vi "Custom Photobleach Length.vi"(8 "Stage Limits":T1={"Y Min"=-inf, "Y Max"=inf, "X Min"=-inf, "X Max"=inf}) -> (0 "Canceled":bool, 1 "Speed (µm/s)":dbl, 2 "Lanes":dbl=1.0, 3 "Length (mm)":dbl)   [LabVIEW 2023]
panel:
  in  "Scan Speed (mm/s):":dbl=0.1 min=0.01 max=1.0
  in  "Number of lanes:":dbl=1.0 min=1.0 step=1.0
  in  "Cancel":bool
  in  "OK":bool
  in  "Lane Length (mm):":dbl=6.0 min=1.0 max=8.0 step=1.0
  # "Please confirm that prism is positioned at the far end\nof the lane. Otherwise microscope WILL BE DAMAGED."
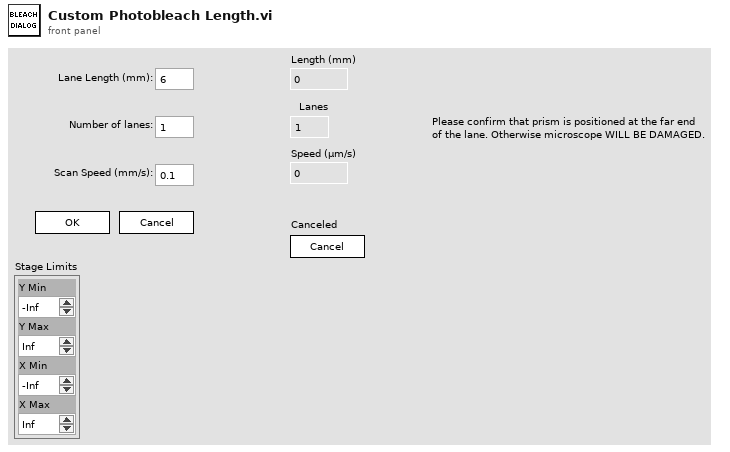
[diagram p1: front panel]
types:
  T1 = cluster{"Y Min":dbl, "Y Max":dbl, "X Min":dbl, "X Max":dbl}
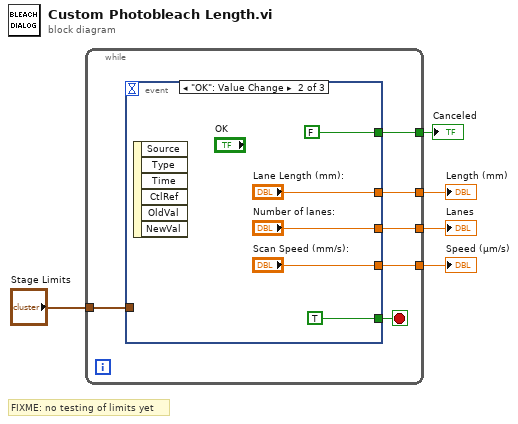
[diagram p0: block diagram]
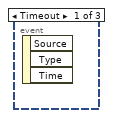
[diagram p2: hidden frame]
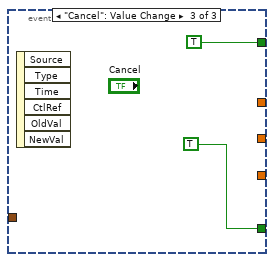
[diagram p3: hidden frame]
diagram:
  # "FIXME: no testing of limits yet"
  n1 = while {
    tunnel: [w10] -> w5
    tunnel: [w9] -> w4
    tunnel: [w8] -> w3
    tunnel: [w7] -> w2
    tunnel: "Stage Limits" -> [w6]
    stop <- w11 stop-if-true
    n2 = event shown="[1] \"OK\": Value Change" {
      selector: _ -> [_ _ _]
      dyn-events: _ -> [_ _ _]
      timeout: _ -> [_ _ _]
      tunnel: [_ TRUE TRUE] -> w11
      tunnel: [_ FALSE TRUE] -> w10
      tunnel: [_ "Lane Length (mm):" _] -> w9
      tunnel: [_ "Number of lanes:" _] -> w8
      tunnel: [_ "Scan Speed (mm/s):" _] -> w7
      tunnel: w6 -> [_ _ _]
      event Timeout {
        n3 = event-data() -> ()  [unwired: 1 in, 3 out]
      }
      event "OK": Value Change {
        n4 = event-data() -> ()  [unwired: 1 in, 6 out]
      }
      event "Cancel": Value Change {
        n5 = event-data() -> ()  [unwired: 1 in, 6 out]
      }
    }
  }
  "Length (mm)" <- w4
  "Canceled" <- w5
  "Lanes" <- w3
  "Speed (µm/s)" <- w2
